vi "LVM_Write.vi"() -> ()   [LabVIEW 2020]
panel:
  out "Waveform Chart":dynamicdata(graph)
  out "ALARMA":bool
  in  "stop":bool
  in  "LIM":dbl
  in  "TEMP":dbl(slide) scale=0.0..100.0
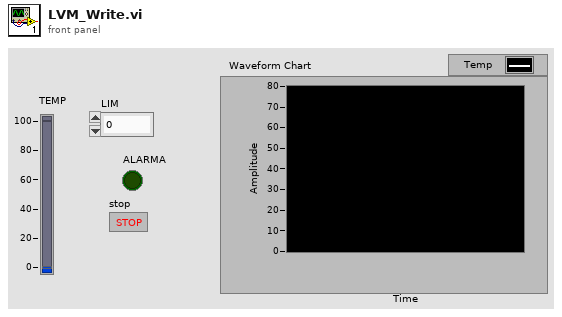
[diagram p1: front panel]
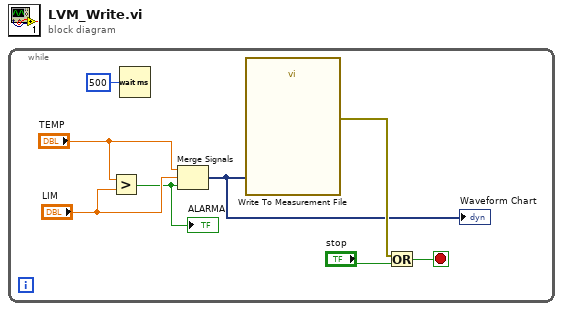
[diagram p0: block diagram]
diagram:
  n1 = while {
    stop <- w4 stop-if-true
    n2 = Greater?(x="TEMP", y="LIM") -> (0:w5:bool)
    "ALARMA" <- w5
    n3 = Wait (ms)(milliseconds to wait=u32 500) -> ()  [unwired: 1 out]
    n4 = Merge Signals("TEMP", "LIM", w5) -> (w1:dynamicdata)
    "Waveform Chart" <- w1
    n5 = call "Write To Measurement File"("Signals"=w1) -> ("error out"=w3:errorcluster)  [unwired: 16 in, 2 out]
    n6 = Or(x=w3, y="stop") -> (x .or. y?=w4:bool)
  }
